vi "subVI_readGPX.vi"(9 "file (use dialog)":path) -> (3 "wpt Array":string[][](array[string]))   [LabVIEW 2019]
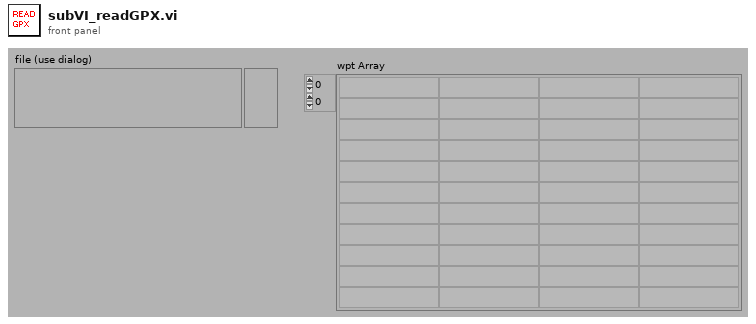
[diagram p1: front panel]
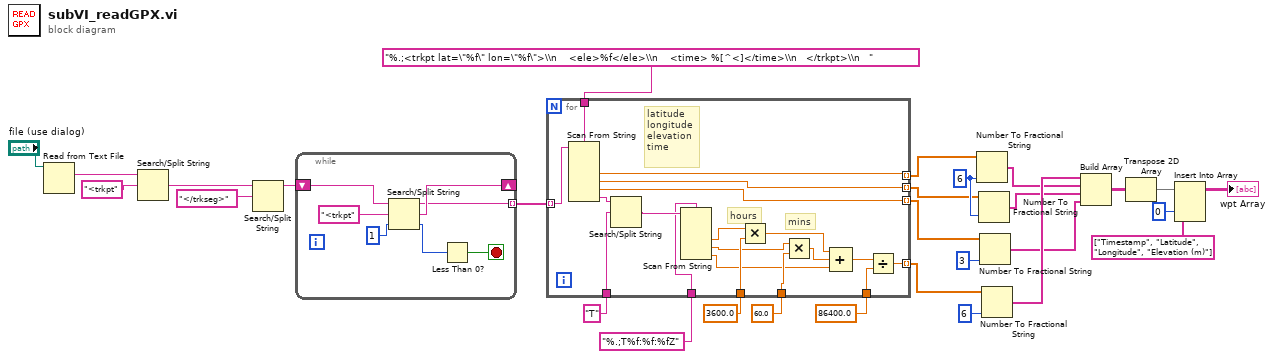
[diagram p0: block diagram]
diagram:
  w22 = i16 6 ("precision (6)")
  n1 = Read from Text File(file (use dialog)="file (use dialog)") -> (text=w29:string)  [unwired: 1 in, 5 out]
  n2 = Search/Split String(string=w29, search string/char (-)="<trkpt") -> (match + rest of string=w26:string)  [unwired: 3 out]
  n3 = Search/Split String(string=w26, search string/char (-)="</trkseg>") -> (substring before match=w25:string)  [unwired: 3 out]
  n4 = while {
    shift-right: [w32] -> _
    shift-left: w25 -> [w33]
    tunnel: [w31] -> w24 mode=indexing
    stop <- w35 stop-if-true
    n5 = Search/Split String(string=w33, search string/char (-)="<trkpt", offset (0)=1) -> (substring before match=w31:string, match + rest of string=w32:string, offset of match=w34:i32)
    n6 = Less Than 0?(x=w34) -> (x < 0?=w35:bool)
  }
  n7 = for {
    tunnel: w24 -> [w55] mode=indexing
    tunnel: [w54] -> w23 mode=indexing
    tunnel: [w53] -> w21 mode=indexing
    tunnel: [w52] -> w20 mode=indexing
    tunnel: "%.;<trkpt lat=\"%f\" lon=\"%f\">\\n    <ele>%f</ele>\\n    <time> %[^<]</time>\\n   </trkpt>\\n   " ("format string") -> [w49]
    tunnel: "T" ("search string/char (-)") -> [w48]
    tunnel: "%.;T%f:%f:%fZ" ("format string") -> [w47]
    tunnel: 3600.0 ("x") -> [w44]
    tunnel: 60.0 ("x") -> [w42]
    tunnel: 86400.0 ("x") -> [w38]
    tunnel: [w37] -> w11 mode=indexing
    # "mins"
    # "hours"
    # "latitude\nlongitude\nelevation\ntime"
    n8 = Scan From String(format string=w49, input string=w55) -> (output 1=w54:dbl, output 2=w53:dbl, output 3=w52:dbl, output 4=w51:string)  [unwired: 2 in, 7 out]
    n9 = Search/Split String(string=w51, search string/char (-)=w48) -> (match + rest of string=w50:string)  [unwired: 3 out]
    n10 = Scan From String(format string=w47, input string=w50) -> (output 1=w45:dbl, output 2=w43:dbl, output 3=w39:dbl)  [unwired: 2 in, 6 out]
    n11 = Multiply(x=w45, y=w44) -> (x*y=w41:dbl)
    n12 = Multiply(x=w43, y=w42) -> (x*y=w40:dbl)
    n13 = Compound Arithmetic op=ADD(w41, w40, w39) -> (w46:dbl)
    n14 = Divide(x=w46, y=w38) -> (x/y=w37:dbl)
  }
  n15 = Number To Fractional String(number=w23, precision (6)=w22) -> (F-format string=w9:string[])  [unwired: 2 in]
  n16 = Number To Fractional String(number=w21, precision (6)=w22) -> (F-format string=w8:string[])  [unwired: 2 in]
  n17 = Number To Fractional String(number=w20, precision (6)=i16 3) -> (F-format string=w7:string[])  [unwired: 2 in]
  n18 = Number To Fractional String(number=w11, precision (6)=i16 6) -> (F-format string=w10:string[])  [unwired: 2 in]
  n19 = Build Array(w10, w9, w8, w7) -> (w5:string[][])
  n20 = Transpose 2D Array(2D array=w5) -> (transposed array=w4:string[][])
  n21 = Insert Into Array(array=w4, index (row)=0, new element=string[] ["Timestamp", "Latitude", "Longitude", "Elevation (m)"]) -> (→"wpt Array":string[][])  [unwired: 1 in]
